vi "Read Warmed-Up State.vi"(8 "error in (no error)":errorcluster, 11 "VISA resource name":refnum<visa-resource-name>) -> (0 "error out":errorcluster, 2 "Warmed-Up":bool, 3 "VISA resource name out":refnum<visa-resource-name>)   [LabVIEW 2018, in "Agilent ENA Series.lvlib"]
doc: "Reads out whether warm-up to satisfy the specifications of the E5070B/E5071B is enough.\n\nNotes:\n(1) This VI is not supported by the E5071C, E5063A or E5080A.\n(2) For the E5071C the instrument always returns TRUE."
uses:
  Agilent ENA Series.lvlib
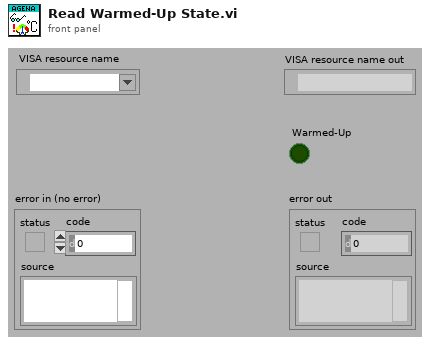
[diagram p1: front panel]
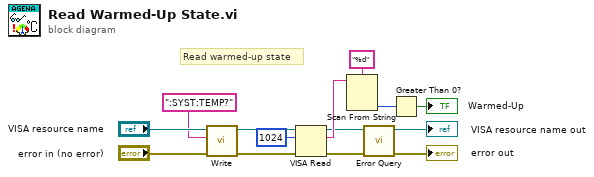
[diagram p0: block diagram]
diagram:
  # "Read warmed-up state"
  n1 = call "Write.vi"("error in (no error)"="error in (no error)", "String ()"=":SYST:TEMP?", "VISA resource name"="VISA resource name") -> ("error out"=w10:errorcluster, "VISA resource name out"=w11:refnum<visa-resource-name>)  [unwired: 6 in, 1 out]
  n2 = VISA Read(VISA resource name=w11, byte count=u32 1024, error in (no error)=w10) -> (VISA resource name out=w4:refnum<visa-resource-name>, read buffer=w8:string, error out=w3:errorcluster)  [unwired: 1 out]
  n3 = Scan From String(format string="%d", input string=w8) -> (output 1=w6:i32)  [unwired: 3 in, 3 out]
  n4 = call "Error Query.vi"("error in (no error)"=w3, "VISA resource name"=w4) -> ("error out"=→"error out":errorcluster, "VISA resource name out"=→"VISA resource name out":refnum<visa-resource-name>)  [unwired: 6 in, 2 out]
  n5 = Greater Than 0?(x=w6) -> (x > 0?=→"Warmed-Up":bool)
